vi "13_2b.vi"() -> ()   [LabVIEW 2018]
panel:
  out "Solution":ext
  in  "Input":string="1000052\n23,x,x,x,x,x,x,x,x,x,x,x,x,x,x,x,x,37,x,x,x,x,x,863,x,x,x,x,x,x,x,x,x,x,x,19,13,x,x,x,17,x,x,x,x,x,x,x,x,x,x,x,29,x,571,x,x,x,x,x,x,x,x,x,x,x,x,x,x,x,x,x,x,x,x,x,x,x,x,x,x,x,x,x,x,x,x,x,x,x,x,x,x,x,x,41"
  # "The earliest timestamp that matches the list 17,x,13,19 is 3417.\n67,7,59,61 first occurs at timestamp 754018.\n67,x,7,59,61 first occurs at timestamp 779210.\n67,7,x,59,61 first occurs at timestamp 1261476.\n1789,37,47,1889 first occurs at timestamp 1202161486."
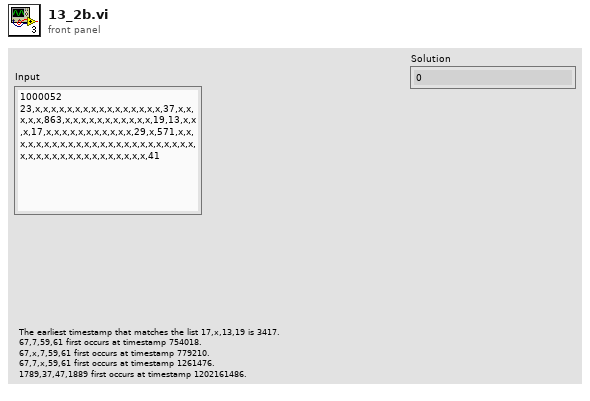
[diagram p1: front panel]
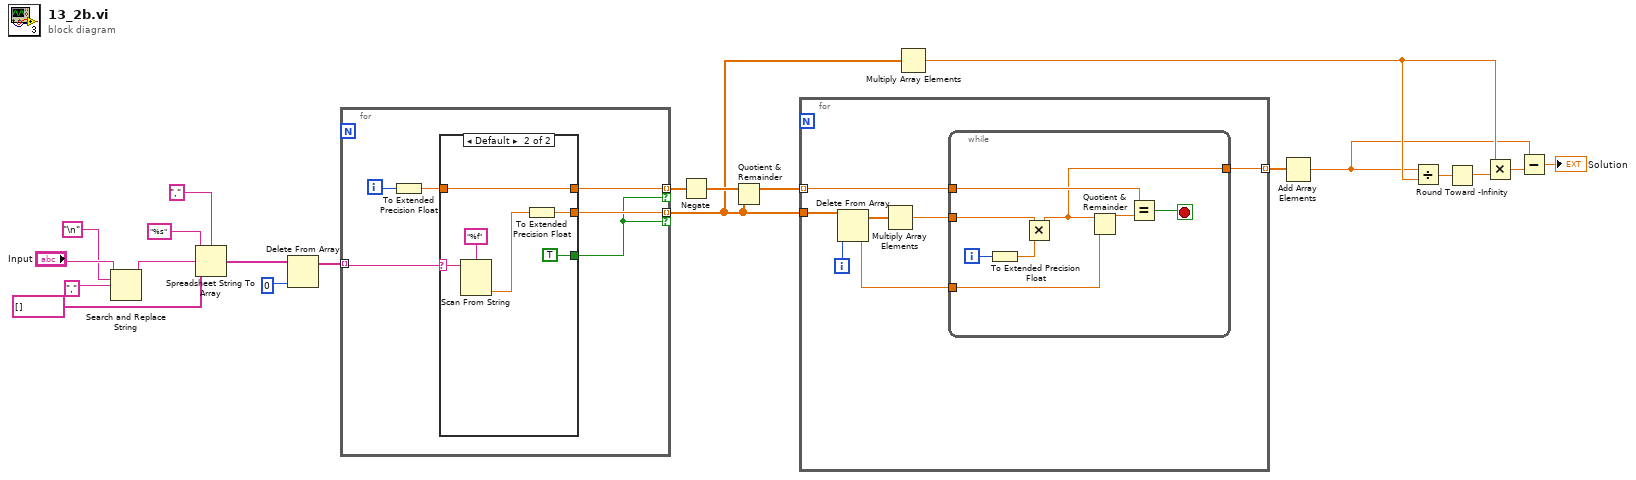
[diagram p0: block diagram]
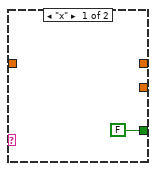
[diagram p2: hidden frame]
diagram:
  n1 = Search and Replace String(input string="Input", search string="\n", replace string=",") -> (result string=w17:string)  [unwired: 5 in, 3 out]
  n2 = Spreadsheet String To Array(delimiter (Tab)=",", format string="%s", spreadsheet string=w17, array type (2D Dbl)=string[] []) -> (array=w14:string[])
  n3 = Delete From Array(array=w14, index=0) -> (array with subset deleted=w12:string[])  [unwired: 1 in, 1 out]
  n4 = for {
    tunnel: w12 -> [w27] mode=indexing
    tunnel: [w25] -> w1 mode=indexing if=w23
    tunnel: [w24] -> w10 mode=indexing if=w23
    i -> [w26]
    n5 = To Extended Precision Float(1:w26) -> (0:w22:ext)
    n6 = case shown="Default" w27 {
      selector: w27 -> [_ w33]
      tunnel: [FALSE TRUE] -> w23
      tunnel: w22 -> [_ w31]
      tunnel: [_ w29] -> w25
      tunnel: [_ w31] -> w24
      frame "x" {
      }
      frame Default {
        n7 = Scan From String(format string="%f", input string=w33) -> (output 1=w30:dbl)  [unwired: 3 in, 3 out]
        n8 = To Extended Precision Float(1:w30) -> (0:w29:ext)
      }
    }
  }
  n9 = Negate(x=w10) -> (-x=w8:ext[])
  n10 = Quotient & Remainder(x=w8, y=w1) -> (x-y*floor(x/y)=w9:ext[])  [unwired: 1 out]
  n11 = for {
    tunnel: w1 -> [w40]
    tunnel: w9 -> [w39] mode=indexing
    tunnel: [w38] -> w11 mode=indexing
    i -> [w41]
    n12 = Delete From Array(array=w40, index=w41) -> (deleted portion=w35:ext, array with subset deleted=w36:ext[])  [unwired: 1 in]
    n13 = Multiply Array Elements(1:w36) -> (0:w37:ext)
    n14 = while {
      tunnel: w37 -> [w46]
      tunnel: w39 -> [w49]
      tunnel: [w44] -> w38
      tunnel: w35 -> [w45]
      i -> [w43]
      stop <- w48 stop-if-true
      n15 = To Extended Precision Float(1:w43) -> (0:w42:ext)
      n16 = Multiply(x=w46, y=w42) -> (x*y=w44:ext)
      n17 = Quotient & Remainder(x=w44, y=w45) -> (x-y*floor(x/y)=w47:ext)  [unwired: 1 out]
      n18 = Equal?(x=w49, y=w47) -> (x = y?=w48:bool)
    }
  }
  n19 = Multiply Array Elements(1:w1) -> (0:w5:ext)
  n20 = Add Array Elements(numeric array=w11) -> (sum=w2:ext)
  n21 = Divide(x=w2, y=w5) -> (x/y=w7:ext)
  n22 = Round Toward -Infinity(1:w7) -> (0:w6:ext)
  n23 = Multiply(x=w5, y=w6) -> (x*y=w4:ext)
  n24 = Subtract(x=w2, y=w4) -> (x-y=→"Solution":ext)
